vi "Read IO_Mode.vi"(8 "error in (no error)":errorcluster, 11 "DIG_IO in":refnum<class "DIG_IO.lvclass">) -> (0 "error out":errorcluster, 2 "IO_Mode":T1, 3 "DIG_IO out":refnum<class "DIG_IO.lvclass">)   [LabVIEW 2019, in "DIG_IO.lvlib" / "DIG_IO.lvclass"]
uses:
  Library/DIG_IO.lvclass
  Custom Controls/IO Mode.ctl
  Library/DIG_IO.lvclass/DIG_IO.ctl
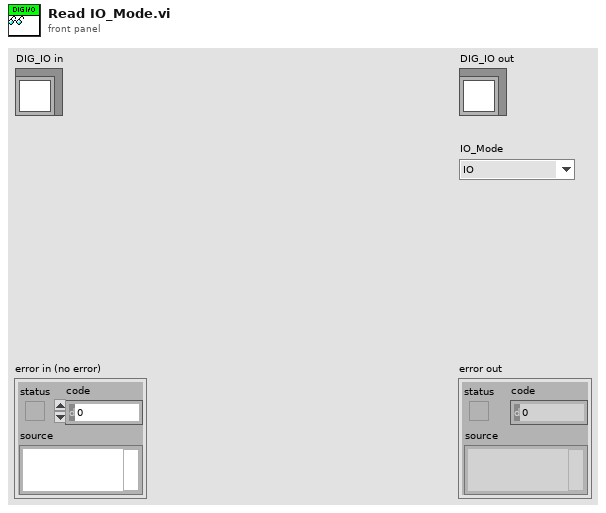
[diagram p1: front panel]
types:
  T1 = typedef "DIG_IO.lvlib/DIG_IO.lvclass/IO Mode.ctl" = enum16{"IO", "IN", "OUT"}
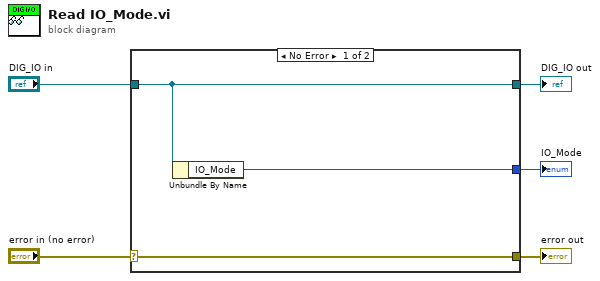
[diagram p0: block diagram]
diagram:
  n1 = case shown="No Error" "error in (no error)" {
    selector: "error in (no error)" -> [w8 w9]
    tunnel: [w8 w9] -> w4
    tunnel: [w7 w10] -> w2
    tunnel: "DIG_IO in" -> [w7 w10]
    tunnel: [w6 _] -> w1
    frame No Error {
      n2 = Unbundle By Name(w7) -> ("IO_Mode"=w6:T1)
    }
    frame Error {
    }
  }
  "error out" <- w4
  "DIG_IO out" <- w2
  "IO_Mode" <- w1
